vi "test_Basic Deployment.vi"(8 "error in (no error)":errorcluster, 11 "DMA Channels Basic Testing in":refnum<class "FPGA Addon DMA Channels Basic System Tests.lvclass">) -> (0 "error out":errorcluster, 3 "DMA Channels Basic Testing out":refnum<class "FPGA Addon DMA Channels Basic System Tests.lvclass">)   [LabVIEW 2020, in "FPGA Addon DMA Channels Basic System Tests.lvclass"]
uses:
  FPGA Addon DMA Channels Basic System Tests.lvclass
  C:/Program Files (x86)/National Instruments/LabVIEW 2020/vi.lib/NI/VeriStand Custom Device Testing Tools/VeriStandTestCase/VeriStandTestCase.lvclass
  <vilib>/NI/VeriStand Custom Device Testing Tools/VeriStandTestUtilities/SystemDefinitionInformation.ctl
  <vilib>/NI/VeriStand Custom Device Testing Tools/VeriStandTestUtilities/TargetInformation.ctl
  <vilib>/NI/VeriStand Custom Device Testing Tools/VeriStandTestUtilities/ChassisInformation.ctl
  <vilib>/NI/VeriStand Custom Device Testing Tools/VeriStandTestUtilities/VeriStandTestUtilities.lvlib
panel:
  out "System Definition Information":T1
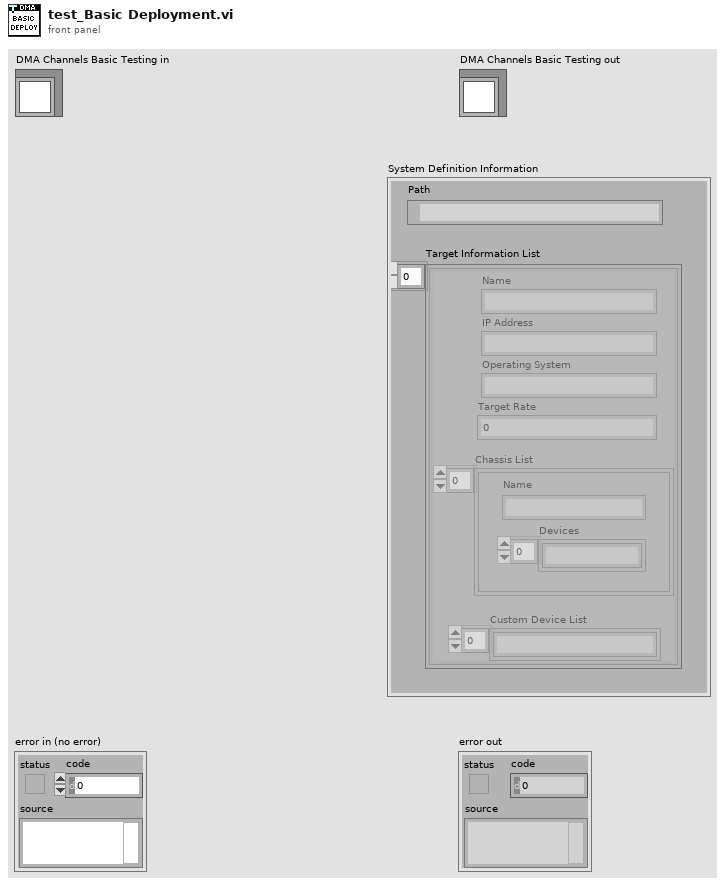
[diagram p1: front panel]
types:
  T1 = typedef "VeriStandTestUtilities.lvlib/SystemDefinitionInformation.ctl" = cluster{"Path":path, "Target Information List":T2[]}
  T2 = typedef "VeriStandTestUtilities.lvlib/TargetInformation.ctl" = cluster{"Name":string, "IP Address":string, "Operating System":string, "Target Rate":dbl, "Chassis List":T3[], "Custom Device List":string[]}
  T3 = typedef "VeriStandTestUtilities.lvlib/ChassisInformation.ctl" = cluster{"Name":string, "Devices":string[]}
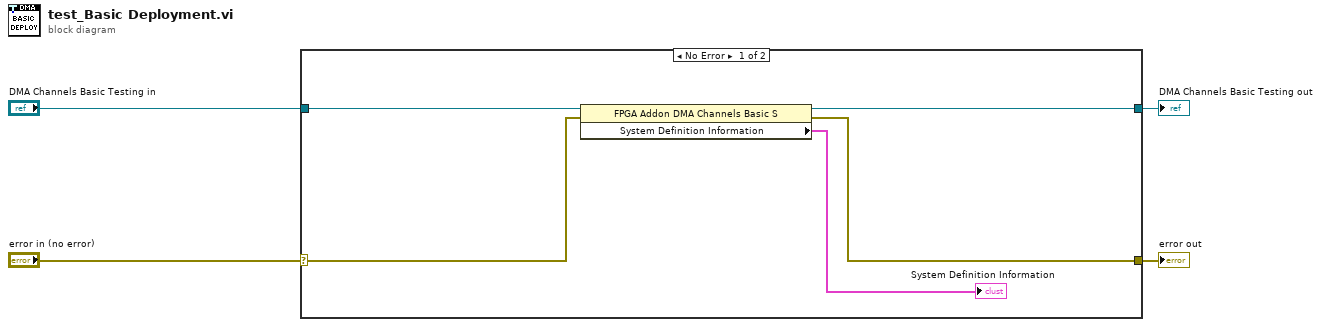
[diagram p0: block diagram]
diagram:
  n1 = case shown="No Error" "error in (no error)" {
    selector: "error in (no error)" -> [w7 w11]
    tunnel: [w5 w11] -> w3
    tunnel: [w6 w10] -> w1
    tunnel: "DMA Channels Basic Testing in" -> [w8 w10]
    frame No Error {
      n2 = property class="FPGA Addon DMA Channels Basic S"(reference=w8, error in=w7) -> (reference out=w6:refnum<class "FPGA Addon DMA Channels Basic System Tests.lvclass">, error out=w5:errorcluster, "System Definition Information"=→"System Definition Information":T1)
    }
    frame Error {
    }
  }
  "error out" <- w3
  "DMA Channels Basic Testing out" <- w1
